vi "开关机和泵subvi.vi"() -> ()   [LabVIEW 2013]
panel:
  in  "Stopprogram":bool
  out "PumpSpeed":u8
  out "PumpTemp":u16
  out "PumpKW":dbl
  out "PumpAmps":dbl
  out "PumpVolts":dbl
  in  "SopPump":bool
  in  "StartPump":bool
  in  "ConfiguredPumpCom":refnum<visa-resource-name>
  in  "Startsystem":bool
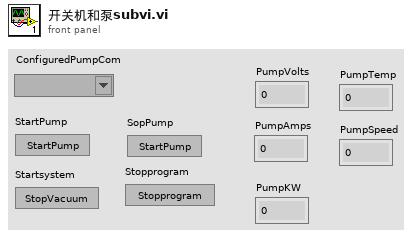
[diagram p1: front panel]
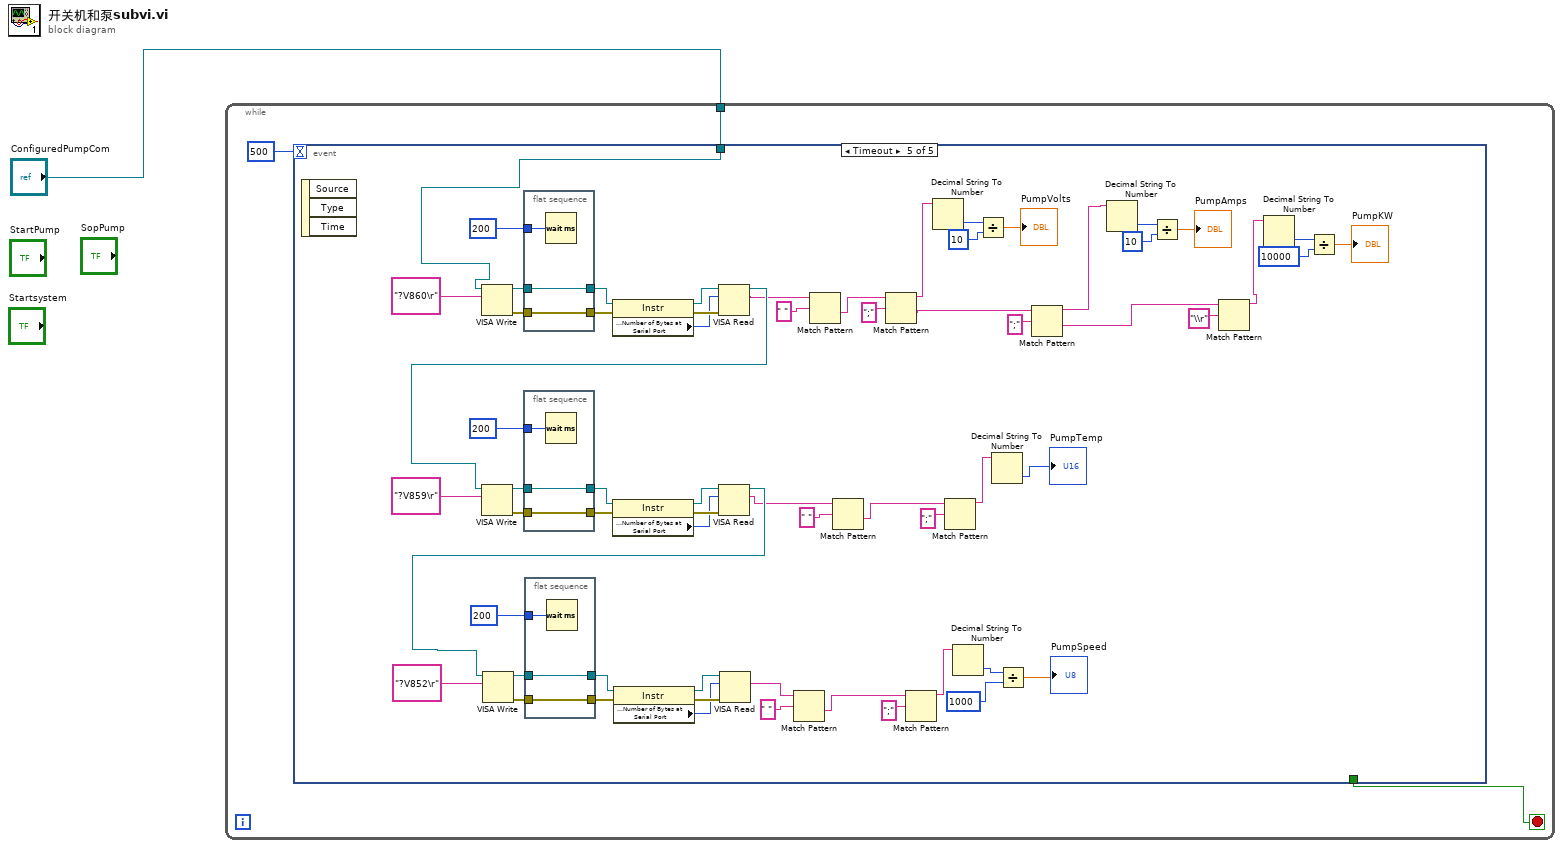
[diagram p0: block diagram]
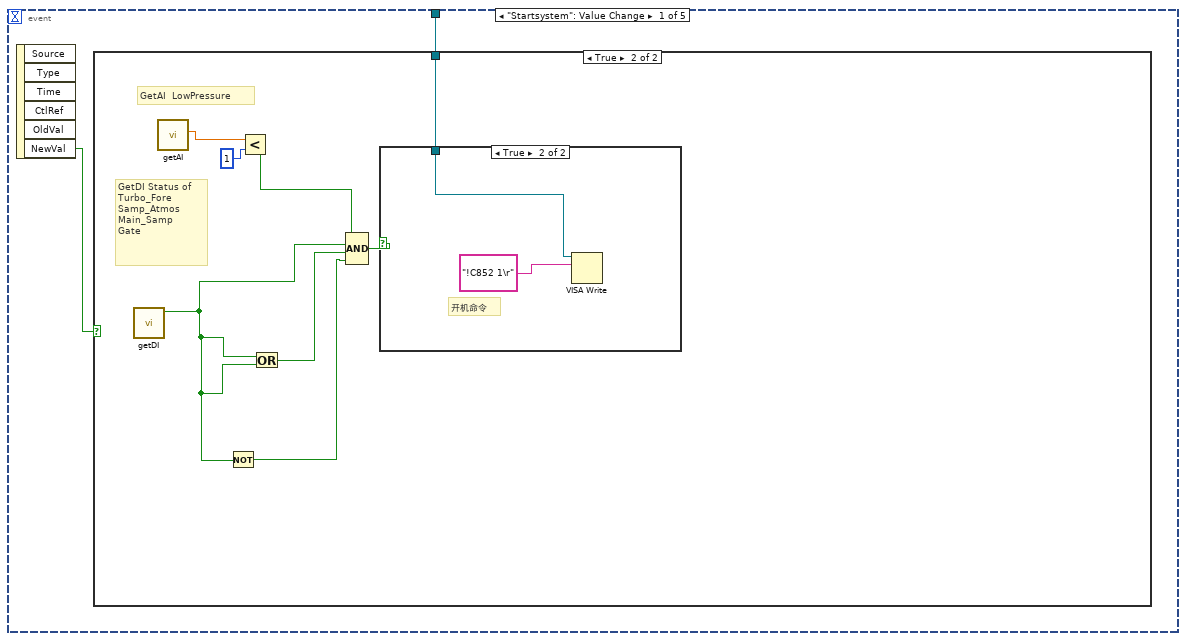
[diagram p2: hidden frame]
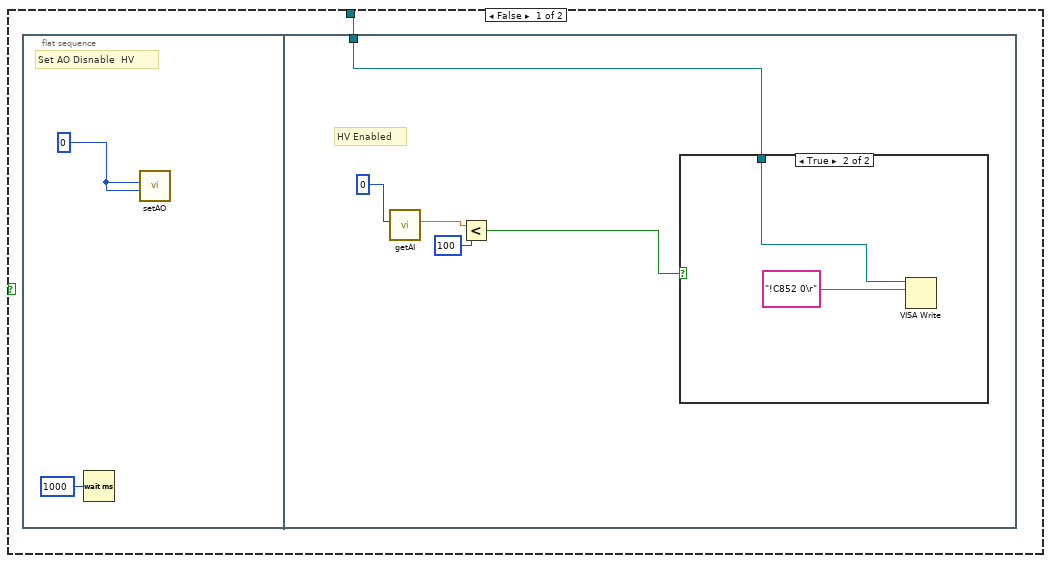
[diagram p3: hidden frame]
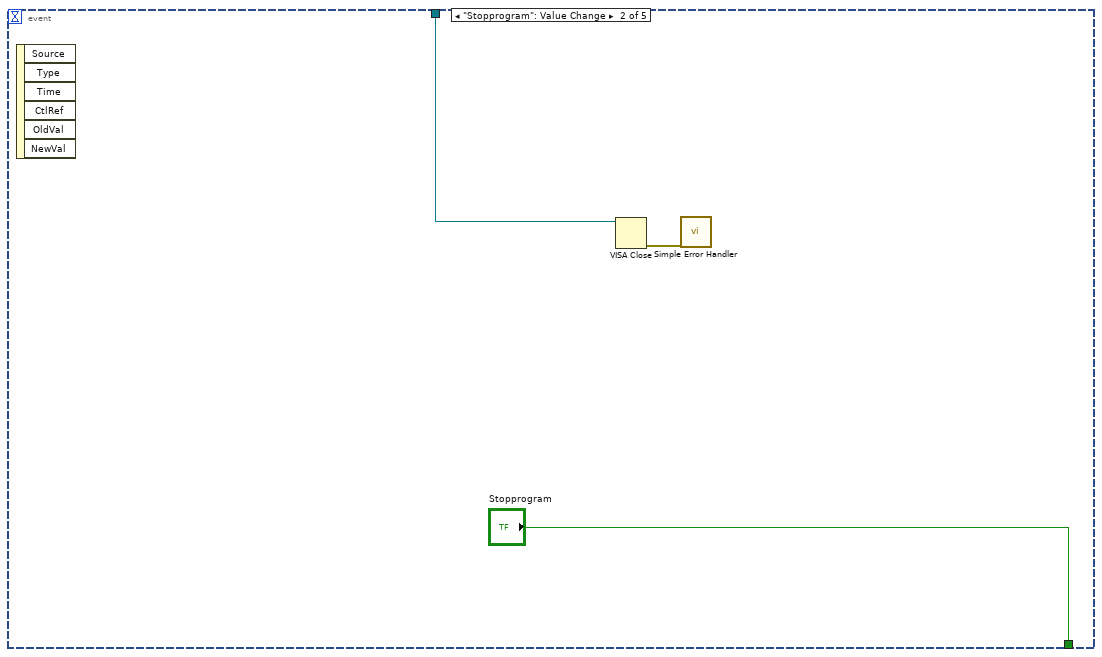
[diagram p6: hidden frame]
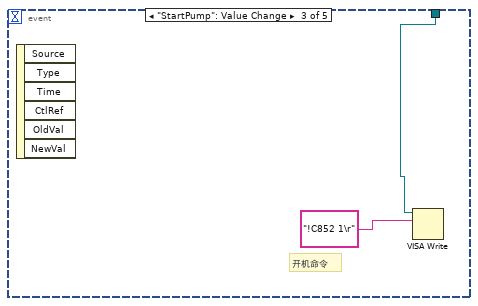
[diagram p7: hidden frame]
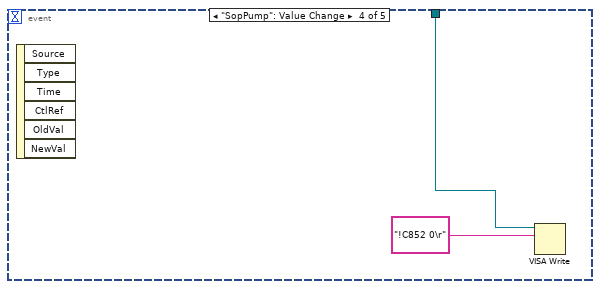
[diagram p8: hidden frame]
diagram:
  n1 = while {
    tunnel: "ConfiguredPumpCom" -> [w2]
    stop <- w3 stop-if-true
    n2 = event shown="[4] Timeout" {
      selector: _ -> [_ _ _ _ _]
      dyn-events: _ -> [_ _ _ _ _]
      timeout: 500 -> [_ _ _ _ _]
      tunnel: [_ "Stopprogram" _ _ _] -> w3
      tunnel: w2 -> [w5 w27 w30 w32 w34]
      event "Startsystem": Value Change {
        n3 = event-data() -> ("NewVal"=w6:bool)  [unwired: 1 in, 5 out]
        n4 = case shown="True" w6 {
          tunnel: w5 -> [w7 w17]
          frame False {
            n5 = flat-sequence {
              tunnel: w7 -> [w14]
              frame #0 {
                w8 = 0
                # "Set AO Disnable  HV"
                n6 = Wait (ms)(milliseconds to wait=u32 1000) -> ()  [unwired: 1 out]
                n7 = call "setAO.vi"("value"=w8, "channel"=w8) -> ()  [unwired: 9 in, 1 out]
              }
              frame #1 {
                # "HV Enabled"
                n8 = call "getAI.vi"("channel"=0) -> ("result"=w12:dbl)  [unwired: 9 in, 1 out]
                n9 = Less?(x=w12, y=100) -> (x < y?=w10:bool)
                n10 = case shown="True" w10 {
                  tunnel: w14 -> [_ w15]
                  frame False {
                  }
                  frame True {
                    n11 = VISA Write(VISA resource name=w15, write buffer="!C852 0\r" ("Command")) -> ()  [unwired: 1 in, 3 out]
                  }
                }
              }
            }
          }
          frame True {
            # "GetAI  LowPressure"
            # "GetDI Status of\nTurbo_Fore\nSamp_Atmos\nMain_Samp\nGate"
            n12 = call "getDI.vi"() -> ("result"=w18:bool)  [unwired: 10 in, 1 out]
            n13 = call "getAI.vi"() -> ("result"=w19:dbl)  [unwired: 10 in, 1 out]
            n14 = Not(x=w18) -> (.not. x?=w20:bool)
            n15 = Less?(x=w19, y=1) -> (x < y?=w23:bool)
            n16 = Or(x=w18, y=w18) -> (x .or. y?=w22:bool)
            n17 = Compound Arithmetic op=AND(w23, w18, w22, w20) -> (w21:bool)
            n18 = case shown="True" w21 {
              tunnel: w17 -> [_ w25]
              frame False {
              }
              frame True {
                # "开机命令"
                n19 = VISA Write(VISA resource name=w25, write buffer="!C852 1\r" ("Command")) -> ()  [unwired: 1 in, 3 out]
              }
            }
          }
        }
      }
      event "Stopprogram": Value Change {
        n20 = event-data() -> ()  [unwired: 1 in, 6 out]
        n21 = VISA Close(VISA resource name=w27) -> (error out=w28:errorcluster)  [unwired: 1 in]
        n22 = call <vilib>:"Simple Error Handler.vi"("error in (no error)"=w28) -> ()  [unwired: 1 in, 8 out]
      }
      event "StartPump": Value Change {
        # "开机命令"
        n23 = event-data() -> ()  [unwired: 1 in, 6 out]
        n24 = VISA Write(VISA resource name=w30, write buffer="!C852 1\r" ("Command")) -> ()  [unwired: 1 in, 3 out]
      }
      event "SopPump": Value Change {
        n25 = event-data() -> ()  [unwired: 1 in, 6 out]
        n26 = VISA Write(VISA resource name=w32, write buffer="!C852 0\r" ("Command")) -> ()  [unwired: 1 in, 3 out]
      }
      event Timeout {
        n27 = event-data() -> ()  [unwired: 1 in, 3 out]
        n28 = VISA Write(VISA resource name=w34, write buffer="?V860\r" ("Command")) -> (VISA resource name out=w41:refnum<visa-resource-name>, error out=w43:errorcluster)  [unwired: 1 in, 1 out]
        n29 = flat-sequence {
          tunnel: w43 -> [w105]
          tunnel: [w105] -> w42
          tunnel: w41 -> [w104]
          tunnel: [w104] -> w40
          tunnel: u32 200 ("delay before read (ms)") -> [w106]
          frame #0 {
            n30 = Wait (ms)(milliseconds to wait=w106) -> ()  [unwired: 1 out]
          }
        }
        n31 = flat-sequence {
          tunnel: w72 -> [w102]
          tunnel: [w102] -> w71
          tunnel: w70 -> [w101]
          tunnel: [w101] -> w69
          tunnel: u32 200 ("delay before read (ms)") -> [w103]
          frame #0 {
            n32 = Wait (ms)(milliseconds to wait=w103) -> ()  [unwired: 1 out]
          }
        }
        n33 = flat-sequence {
          tunnel: w88 -> [w99]
          tunnel: [w99] -> w87
          tunnel: w86 -> [w98]
          tunnel: [w98] -> w85
          tunnel: u32 200 ("delay before read (ms)") -> [w100]
          frame #0 {
            n34 = Wait (ms)(milliseconds to wait=w100) -> ()  [unwired: 1 out]
          }
        }
        n35 = property class="Instr"(reference=w40, error in=w42) -> (reference out=w38:refnum<visa-resource-name>, error out=w37:errorcluster, "Serial Settings:Number of Bytes at Serial Port"=w36:u32)
        n36 = property class="Instr"(reference=w69, error in=w71) -> (reference out=w67:refnum<visa-resource-name>, error out=w66:errorcluster, "Serial Settings:Number of Bytes at Serial Port"=w65:u32)
        n37 = property class="Instr"(reference=w85, error in=w87) -> (reference out=w83:refnum<visa-resource-name>, error out=w82:errorcluster, "Serial Settings:Number of Bytes at Serial Port"=w81:u32)
        n38 = VISA Read(VISA resource name=w38, byte count=w36, error in (no error)=w37) -> (VISA resource name out=w73:refnum<visa-resource-name>, read buffer=w53:string)  [unwired: 2 out]
        n39 = VISA Write(VISA resource name=w73, write buffer="?V859\r" ("Command")) -> (VISA resource name out=w70:refnum<visa-resource-name>, error out=w72:errorcluster)  [unwired: 1 in, 1 out]
        n40 = VISA Read(VISA resource name=w67, byte count=w65, error in (no error)=w66) -> (VISA resource name out=w89:refnum<visa-resource-name>, read buffer=w78:string)  [unwired: 2 out]
        n41 = VISA Write(VISA resource name=w89, write buffer="?V852\r" ("Command")) -> (VISA resource name out=w86:refnum<visa-resource-name>, error out=w88:errorcluster)  [unwired: 1 in, 1 out]
        n42 = VISA Read(VISA resource name=w83, byte count=w81, error in (no error)=w82) -> (read buffer=w94:string)  [unwired: 3 out]
        n43 = Match Pattern(string=w94, regular expression=" ") -> (after substring=w91:string)  [unwired: 1 in, 3 out]
        n44 = Match Pattern(string=w53, regular expression=" ") -> (after substring=w55:string)  [unwired: 1 in, 3 out]
        n45 = Match Pattern(string=w78, regular expression=" ") -> (after substring=w75:string)  [unwired: 1 in, 3 out]
        n46 = Match Pattern(string=w55, regular expression=";") -> (before substring=w57:string, after substring=w59:string)  [unwired: 1 in, 2 out]
        n47 = Match Pattern(string=w91, regular expression=";") -> (before substring=w93:string)  [unwired: 1 in, 3 out]
        n48 = Decimal String To Number(string=w57) -> (number=w44:i32)  [unwired: 2 in, 1 out]
        n49 = Match Pattern(string=w75, regular expression=";") -> (before substring=w77:string)  [unwired: 1 in, 3 out]
        n50 = Decimal String To Number(string=w93) -> (number=w95:i32)  [unwired: 2 in, 1 out]
        n51 = Divide(x=w44, y=10) -> (x/y=→"PumpVolts":dbl)
        n52 = Decimal String To Number(string=w77) -> (number=→"PumpTemp":i32)  [unwired: 2 in, 1 out]
        n53 = Divide(x=w95, y=1000) -> (x/y=→"PumpSpeed":dbl)
        n54 = Match Pattern(string=w59, regular expression=";") -> (before substring=w60:string, after substring=w62:string)  [unwired: 1 in, 2 out]
        n55 = Decimal String To Number(string=w60) -> (number=w47:i32)  [unwired: 2 in, 1 out]
        n56 = Divide(x=w47, y=10) -> (x/y=→"PumpAmps":dbl)
        n57 = Match Pattern(string=w62, regular expression="\\r") -> (before substring=w63:string)  [unwired: 1 in, 3 out]
        n58 = Decimal String To Number(string=w63) -> (number=w50:i32)  [unwired: 2 in, 1 out]
        n59 = Divide(x=w50, y=10000) -> (x/y=→"PumpKW":dbl)
      }
    }
  }
